vi "Individual Relay.vi"(8 "error in (no error)":errorcluster, 9 "relay action":i32(ring)=21 caption="Relay Action" items=["Open Relay"=20, "Close Relay"=21], 10 "relay name":string="k0" caption="Relay Name", 11 "PXIe 2737 in":refnum<class "PXIe 2737.lvclass">) -> (0 "error out":errorcluster, 3 "PXIe 2737 out":refnum<class "PXIe 2737.lvclass">)   [LabVIEW 2021, in "S-Matrix.lvlib" / "PXIe 2737.lvclass"]
uses:
  PXIe 2737.lvclass
  Abstract/Abstract.lvclass
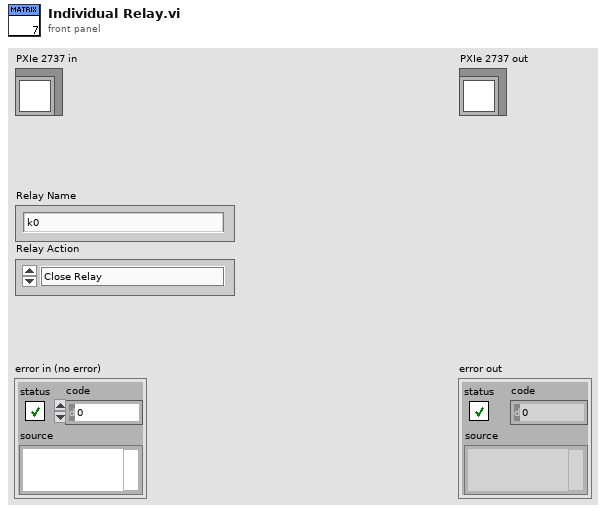
[diagram p1: front panel]
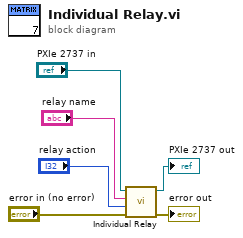
[diagram p0: block diagram]
diagram:
  n1 = call-parent "Individual Relay.vi"("error in (no error)"="error in (no error)", "relay action"="relay action", "relay name"="relay name", "Abstract in"="PXIe 2737 in") -> ("error out"=→"error out":errorcluster, "Abstract out"=→"PXIe 2737 out":refnum<class "PXIe 2737.lvclass">)  [unwired: 6 in]
